vi "Periodic Tasks.vi"(8 "error in":errorcluster) -> ()   [LabVIEW 2013]
doc: "This VI runs in parallel to other tasks. It can contain as many user-defined periodic loops as you need. These can carry out PID or other sorts of timed response."
uses:
  <vilib>/Rock Robotics/SystemInterfaces/Utilities/FPGA_UtilitiesLED Source.ctl
  <vilib>/Rock Robotics/SystemInterfaces/Utilities/FPGA_UtilitiesLED State.ctl
  Robot Global Data.vi
  <vilib>/Rock Robotics/WPI/Compressor/WPI_CompressorGetSetRefNum.vi
  Systems/Drive/Drive Global.vi
  Systems/Cannon/Cannon Global.vi
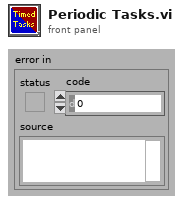
[diagram p1: front panel]
types:
  T1 = typedef "FPGA_UtilitiesLED State.ctl" = enum16{"Off", "On", "Toggle"}
  T2 = typedef "FPGA_UtilitiesLED Source.ctl" = enum16{"User LED", "FPGA LED"}
  T3 = typedef "WPI_CompressorDevRef.ctl" = cluster{"DevStatus":errorcluster, "DigitalInputDevRef":T4, "RelayDevRef":T7}
  T4 = typedef "WPI_DigitalInputDevRef.ctl" = cluster{"DevStatus":errorcluster, "DIO Channel":T5, "Digital Module":T6}
  T5 = typedef "FPGA_DIOChannel.ctl" = enum8{"DIO 1", "DIO 2", "DIO 3", "DIO 4", "DIO 5", "DIO 6", "DIO 7", "DIO 8", "DIO 9", "DIO 10", "DIO 11", "DIO 12", "DIO 13", "DIO 14", "Invalid"}
  T6 = typedef "FPGA_TypedefDigitalModule.ctl" = enum16{"Digital Module 1", "Digital Module 2"}
  T7 = typedef "WPI_RelayDevRef.ctl" = cluster{"DevStatus":errorcluster, "Relay Channel":T8, "Digital Module":T6, "Relay Direction":T9}
  T8 = typedef "FPGA_DIORelayChannel.ctl" = enum8{"Relay 1", "Relay 2", "Relay 3", "Relay 4", "Relay 5", "Relay 6", "Relay 7", "Relay 8", "Invalid"}
  T9 = typedef "WPI_RelayDirection.ctl" = enum16{"Both directions", "Forward only", "Reverse only"}
  T10 = typedef "WPI_AnalogChannelDevRef.ctl" = cluster{"DevStatus":errorcluster, "Analog Module":T11, "Analog Channel":T12}
  T11 = typedef "FPGA_TypedefAnalogModule.ctl" = enum16{"Analog Module 1", "Analog Module 2"}
  T12 = typedef "FPGA_AIChannel.ctl" = enum8{"AI 1", "AI 2", "AI 3", "AI 4", "AI 5", "AI 6", "AI 7", "AI 8", "Invalid"}
  T13 = typedef "WPI_EncoderDevRef.ctl" = cluster{"DevStatus":errorcluster, "EncoderIndex":T14, "CounterIndex":T15, "DistancePerCount":dbl, "Decoding Type":T16}
  T14 = typedef "FPGA_EncoderIdx.ctl" = enum8{"Enc 0", "Enc 1", "Enc 2", "Enc 3", "Invalid"}
  T15 = typedef "FPGA_CounterCtrSystemIndex.ctl" = enum8{"Ctr 0", "Ctr 1", "Ctr 2", "Ctr 3", "Ctr 4", "Ctr 5", "Ctr 6", "Ctr 7", "Invalid"}
  T16 = typedef "WPI_EncoderType.ctl" = enum16{"1x", "2x", "4x"}
  T17 = typedef "WPI_SolenoidValue.ctl" = enum16{"Off", "On", "Forward", "Reverse"}
  T18 = cluster{"V - Bus out":dbl, "Manual Power In":dbl, "Stop Auto?":bool, "Ball":bool, "Catch":bool, "Low Point":bool, "Catcher":T17, "Change Catcher?":bool}
  T19 = cluster{"X - Axis":dbl, "Y - Axis":dbl, "Slow Drive?":bool, "Right Side RPM":dbl, "Right Side Distance":dbl, "Left Side RPM ":dbl, "Left Side Distance":dbl}
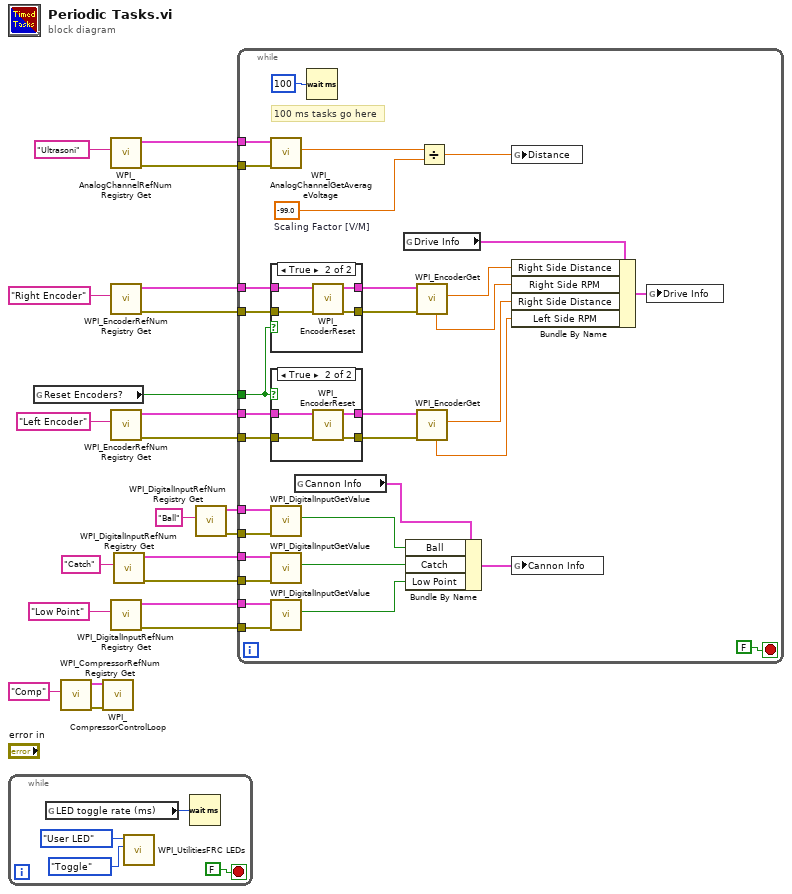
[diagram p0: block diagram]
diagram:
  n1 = while {
    stop <- FALSE stop-if-true
    n2 = global read "Robot Global Data.vi" "LED toggle rate (ms)"() -> (w23:u32)
    n3 = call <vilib>:"WPI_UtilitiesFRC LEDs.vi"("State"=FPGA_UtilitiesLED_State."Toggle", "LED Type"=FPGA_UtilitiesLED_Source."User LED") -> ()  [unwired: 1 in, 9 out]
    n4 = Wait (ms)(milliseconds to wait=w23) -> ()  [unwired: 1 out]
  }
  n5 = global read "Robot Global Data.vi" "Reset Encoders?"() -> (w16:bool)
  n6 = call <vilib>:"WPI_CompressorRefNum Registry Get.vi"("refnum name"="Comp") -> ("error out"=w11:errorcluster, "CompressorDevRef"=w10:T3)  [unwired: 9 in]
  n7 = call <vilib>:"WPI_CompressorControlLoop.vi"("error in (no error)"=w11, "CompressorDevRef"=w10) -> ()  [unwired: 10 in]
  n8 = call <vilib>:"WPI_AnalogChannelRefNum Registry Get.vi"("refnum name"="Ultrasoni") -> ("error out"=w13:errorcluster, "AIDeviceRef"=w14:T10)  [unwired: 9 in]
  n9 = call <vilib>:"WPI_EncoderRefNum Registry Get.vi"("refnum name"="Right Encoder") -> ("error out"=w19:errorcluster, "EncoderDevRef"=w20:T13)  [unwired: 9 in]
  n10 = call <vilib>:"WPI_EncoderRefNum Registry Get.vi"("refnum name"="Left Encoder") -> ("error out"=w21:errorcluster, "EncoderDevRef"=w22:T13)  [unwired: 9 in]
  n11 = call <vilib>:"WPI_DigitalInputRefNum Registry Get.vi"("refnum name"="Low Point") -> ("error out"=w2:errorcluster, "DigitalInputDevRef"=w1:T4)  [unwired: 9 in]
  n12 = call <vilib>:"WPI_DigitalInputRefNum Registry Get.vi"("refnum name"="Catch") -> ("error out"=w4:errorcluster, "DigitalInputDevRef"=w3:T4)  [unwired: 9 in]
  n13 = call <vilib>:"WPI_DigitalInputRefNum Registry Get.vi"("refnum name"="Ball") -> ("error out"=w5:errorcluster, "DigitalInputDevRef"=w6:T4)  [unwired: 9 in]
  n14 = while {
    tunnel: w22 -> [w53]
    tunnel: w21 -> [w52]
    tunnel: w20 -> [w57]
    tunnel: w19 -> [w56]
    tunnel: w16 -> [w49]
    tunnel: w14 -> [w42]
    tunnel: w13 -> [w41]
    tunnel: w6 -> [w37]
    tunnel: w5 -> [w36]
    tunnel: w4 -> [w35]
    tunnel: w3 -> [w34]
    tunnel: w2 -> [w33]
    tunnel: w1 -> [w32]
    stop <- FALSE stop-if-true
    w39 = -99.0  # Scaling Factor [V/M]
    # "100 ms tasks go here"
    n15 = call <vilib>:"WPI_AnalogChannelGetAverageVoltage.vi"("error in (no error)"=w41, "AIDeviceRef"=w42) -> ("Voltage"=w40:dbl)  [unwired: 7 in, 2 out]
    n16 = case shown="True" w49 {
      tunnel: w57 -> [w67 w71]
      tunnel: w56 -> [w66 w70]
      tunnel: [w67 w69] -> w55
      tunnel: [w66 w68] -> w54
      frame False {
      }
      frame True {
        n17 = call <vilib>:"WPI_EncoderReset.vi"("error in (no error)"=w70, "EncoderDevRef"=w71) -> ("error out"=w68:errorcluster, "EncoderDevRef"=w69:T13)  [unwired: 8 in]
      }
    }
    n18 = case shown="True" w49 {
      tunnel: w53 -> [w61 w65]
      tunnel: w52 -> [w60 w64]
      tunnel: [w61 w62] -> w50
      tunnel: [w60 w63] -> w51
      frame False {
      }
      frame True {
        n19 = call <vilib>:"WPI_EncoderReset.vi"("error in (no error)"=w64, "EncoderDevRef"=w65) -> ("error out"=w63:errorcluster, "EncoderDevRef"=w62:T13)  [unwired: 8 in]
      }
    }
    n20 = call <vilib>:"WPI_DigitalInputGetValue.vi"("error in (no error)"=w36, "DigitalInputDevRef"=w37) -> ("Value"=w28:bool)  [unwired: 7 in, 2 out]
    n21 = call <vilib>:"WPI_DigitalInputGetValue.vi"("error in (no error)"=w35, "DigitalInputDevRef"=w34) -> ("Value"=w29:bool)  [unwired: 7 in, 2 out]
    n22 = call <vilib>:"WPI_DigitalInputGetValue.vi"("error in (no error)"=w33, "DigitalInputDevRef"=w32) -> ("Value"=w30:bool)  [unwired: 7 in, 2 out]
    n23 = global read "Cannon Global.vi" "Cannon Info"() -> (w31:T18)
    n24 = Wait (ms)(milliseconds to wait=u32 100) -> ()  [unwired: 1 out]
    n25 = global read "Drive Global.vi" "Drive Info"() -> (w47:T19)
    n26 = Bundle By Name(cluster=w31, "Ball"=w28, "Catch"=w29, "Low Point"=w30) -> (w27:T18)
    n27 = call <vilib>:"WPI_EncoderGet.vi"("error in (no error)"=w54, "EncoderDevRef"=w55) -> ("Distance"=w45:dbl, "Rate"=w46:dbl)  [unwired: 4 in, 4 out]
    n28 = call <vilib>:"WPI_EncoderGet.vi"("error in (no error)"=w51, "EncoderDevRef"=w50) -> ("Distance"=w44:dbl, "Rate"=w43:dbl)  [unwired: 4 in, 4 out]
    n29 = Divide(x=w40, y=w39) -> (x/y=w38:dbl)
    n30 = global write "Robot Global Data.vi" "Distance"(w38) -> ()
    n31 = Bundle By Name(cluster=w47, "Right Side Distance"=w45, "Right Side RPM"=w46, "Right Side Distance"=w44, "Left Side RPM"=w43) -> (w48:T19)
    n32 = global write "Cannon Global.vi" "Cannon Info"(w27) -> ()
    n33 = global write "Drive Global.vi" "Drive Info"(w48) -> ()
  }
